vi "clearBit.vi"(10 "n":i32=-1, 11 "input":u8 format="%08b") -> (3 "output":u8 format="%08b")   [LabVIEW 2013, in "bitwiseOps.lvlib"]
uses:
  bitwiseOps.lvlib
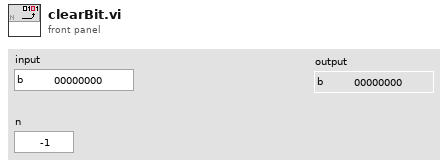
[diagram p1: front panel]
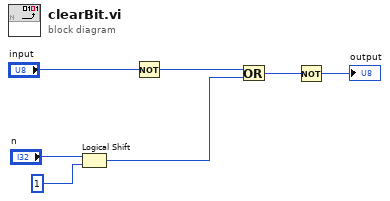
[diagram p0: block diagram]
diagram:
  n1 = Logical Shift(y="n", x=u8 1) -> (x << y=w6:u8)
  n2 = Not(x="input") -> (.not. x?=w3:u8)
  n3 = Or(x=w3, y=w6) -> (x .or. y?=w2:u8)
  n4 = Not(x=w2) -> (.not. x?=→"output":u8)
